vi "BioFeedback19(Adjustable_View).vi"() -> ()   [LabVIEW 2016]
doc: "Use this template to build a producer/consumer design pattern. Use this template when you need to execute a process, such as data analysis, when a data source, such as a triggered acquisition, produces data at an uneven rate and you need to execute the process when the data becomes available."
uses:
  customSubVIs/8ChanWfmArray.ctl
  <vilib>/Utility/file.llb/Write Delimited Spreadsheet (string).vi
  <vilib>/Waveform/WDTFileIO.llb/Export Waveforms To Spreadsheet File (1D).vi
panel:
  in  "log filepath":path
  out "TrialStartTime":timestamp
  in  "Trial Duration":dbl=3.0
  out "Trial Number":dbl
  in  "Session Name":string="Test"
  out "loopTime":dbl=30.0 caption="Upper Cut-Off"
  in  "trial display data":path
  out "Disp Data":cluster{"queue out":refnum<queue>, dbl, dbl}[](array[cluster])
  in  "Target Percentage":dbl=10.0
  out "DisplayActivation":dbl
  out "DisplayBarActivation":dbl(slide) caption="Percent Activation" max=1.0 scale=0.0..100.0
  in  "Display Channel":dbl=0.5
  out "MVC Data":cluster{"queue out":refnum<queue>, dbl, dbl}[](array[cluster])
  out "Trial Name":string="Test"
  in  "Data Directory":path=path "C:/Users/Tinggroup/Desktop/VRMuscleActivationVisualizer/LabviewFiles/Data"
  out "GetMaxStartTime":timestamp
  in  "MVC Number":dbl=1.0
  in  "SecondsToAcquireMax":dbl=3.0
  in  "Frames Per Second":dbl=30.0 caption="Upper Cut-Off"
  in  "EMG Input Device\nProduct Type":string="USB-6009"
  out "raw data":dynamicdata(graph)
  out "dispSize":dbl=20.0 caption="Lower Cut-Off"
  out "mvcSize":dbl=300.0 caption="Upper Cut-Off"
  in  "MVC Window Size (s)":dbl=0.5
  in  "Display Window Size (s)":dbl=0.5
  in  "MVC Raw Path":path
  in  "trial raw data":path
  in  "trial filtered data":path
  in  "MVC Filtered Path":path
  in  "Sample rate (Hz)":dbl=1000.0 caption="Upper Cut-Off"
  out "fps":dbl=20.0 caption="Lower Cut-Off"
  out "rate":dbl=300.0 caption="Upper Cut-Off"
  in  "Set Parameters":bool
  out "lower":dbl=20.0 caption="Lower Cut-Off"
  out "upper":dbl=300.0 caption="Upper Cut-Off"
  in  "Lower Cut-Off":dbl=20.0
  in  "Upper Cut-Off":dbl=500.0
  in  "Mark":bool
  in  "End Trial":bool
  in  "Reset MVC":bool
  in  "Get MVC":bool
  in  "StartTrial":bool
  out "State":T1(ring)
  out "FilteredAndRectified":waveform(dbl)[](graph) caption="Filtered and Rectified"
  in  "stop":bool
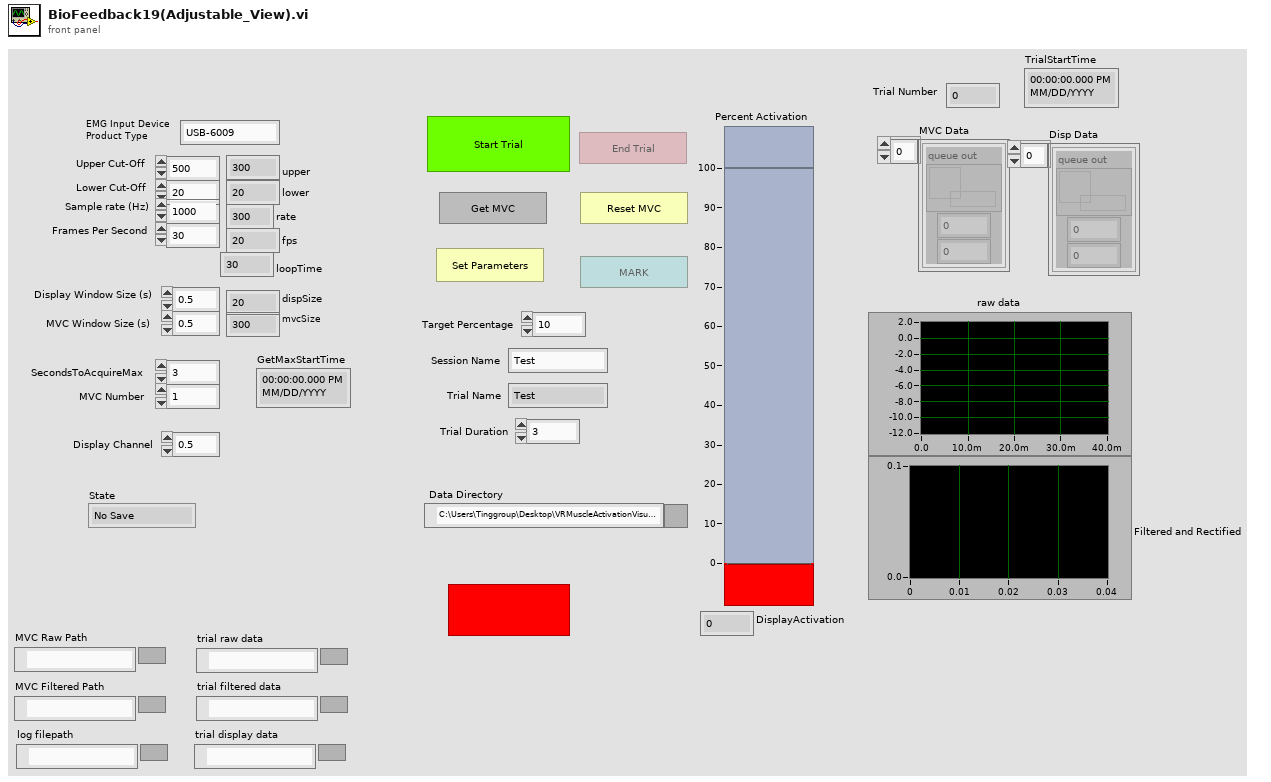
[diagram p1: front panel]
types:
  T1 = enum16{"No Save", "Acquiring Max", "Trial In Progress"}
  T2 = typedef "8ChanWfmArray.ctl" = waveform(dbl)[]
  T3 = enum8{"Enabled", "Disabled", "Disabled and Grayed Out"}
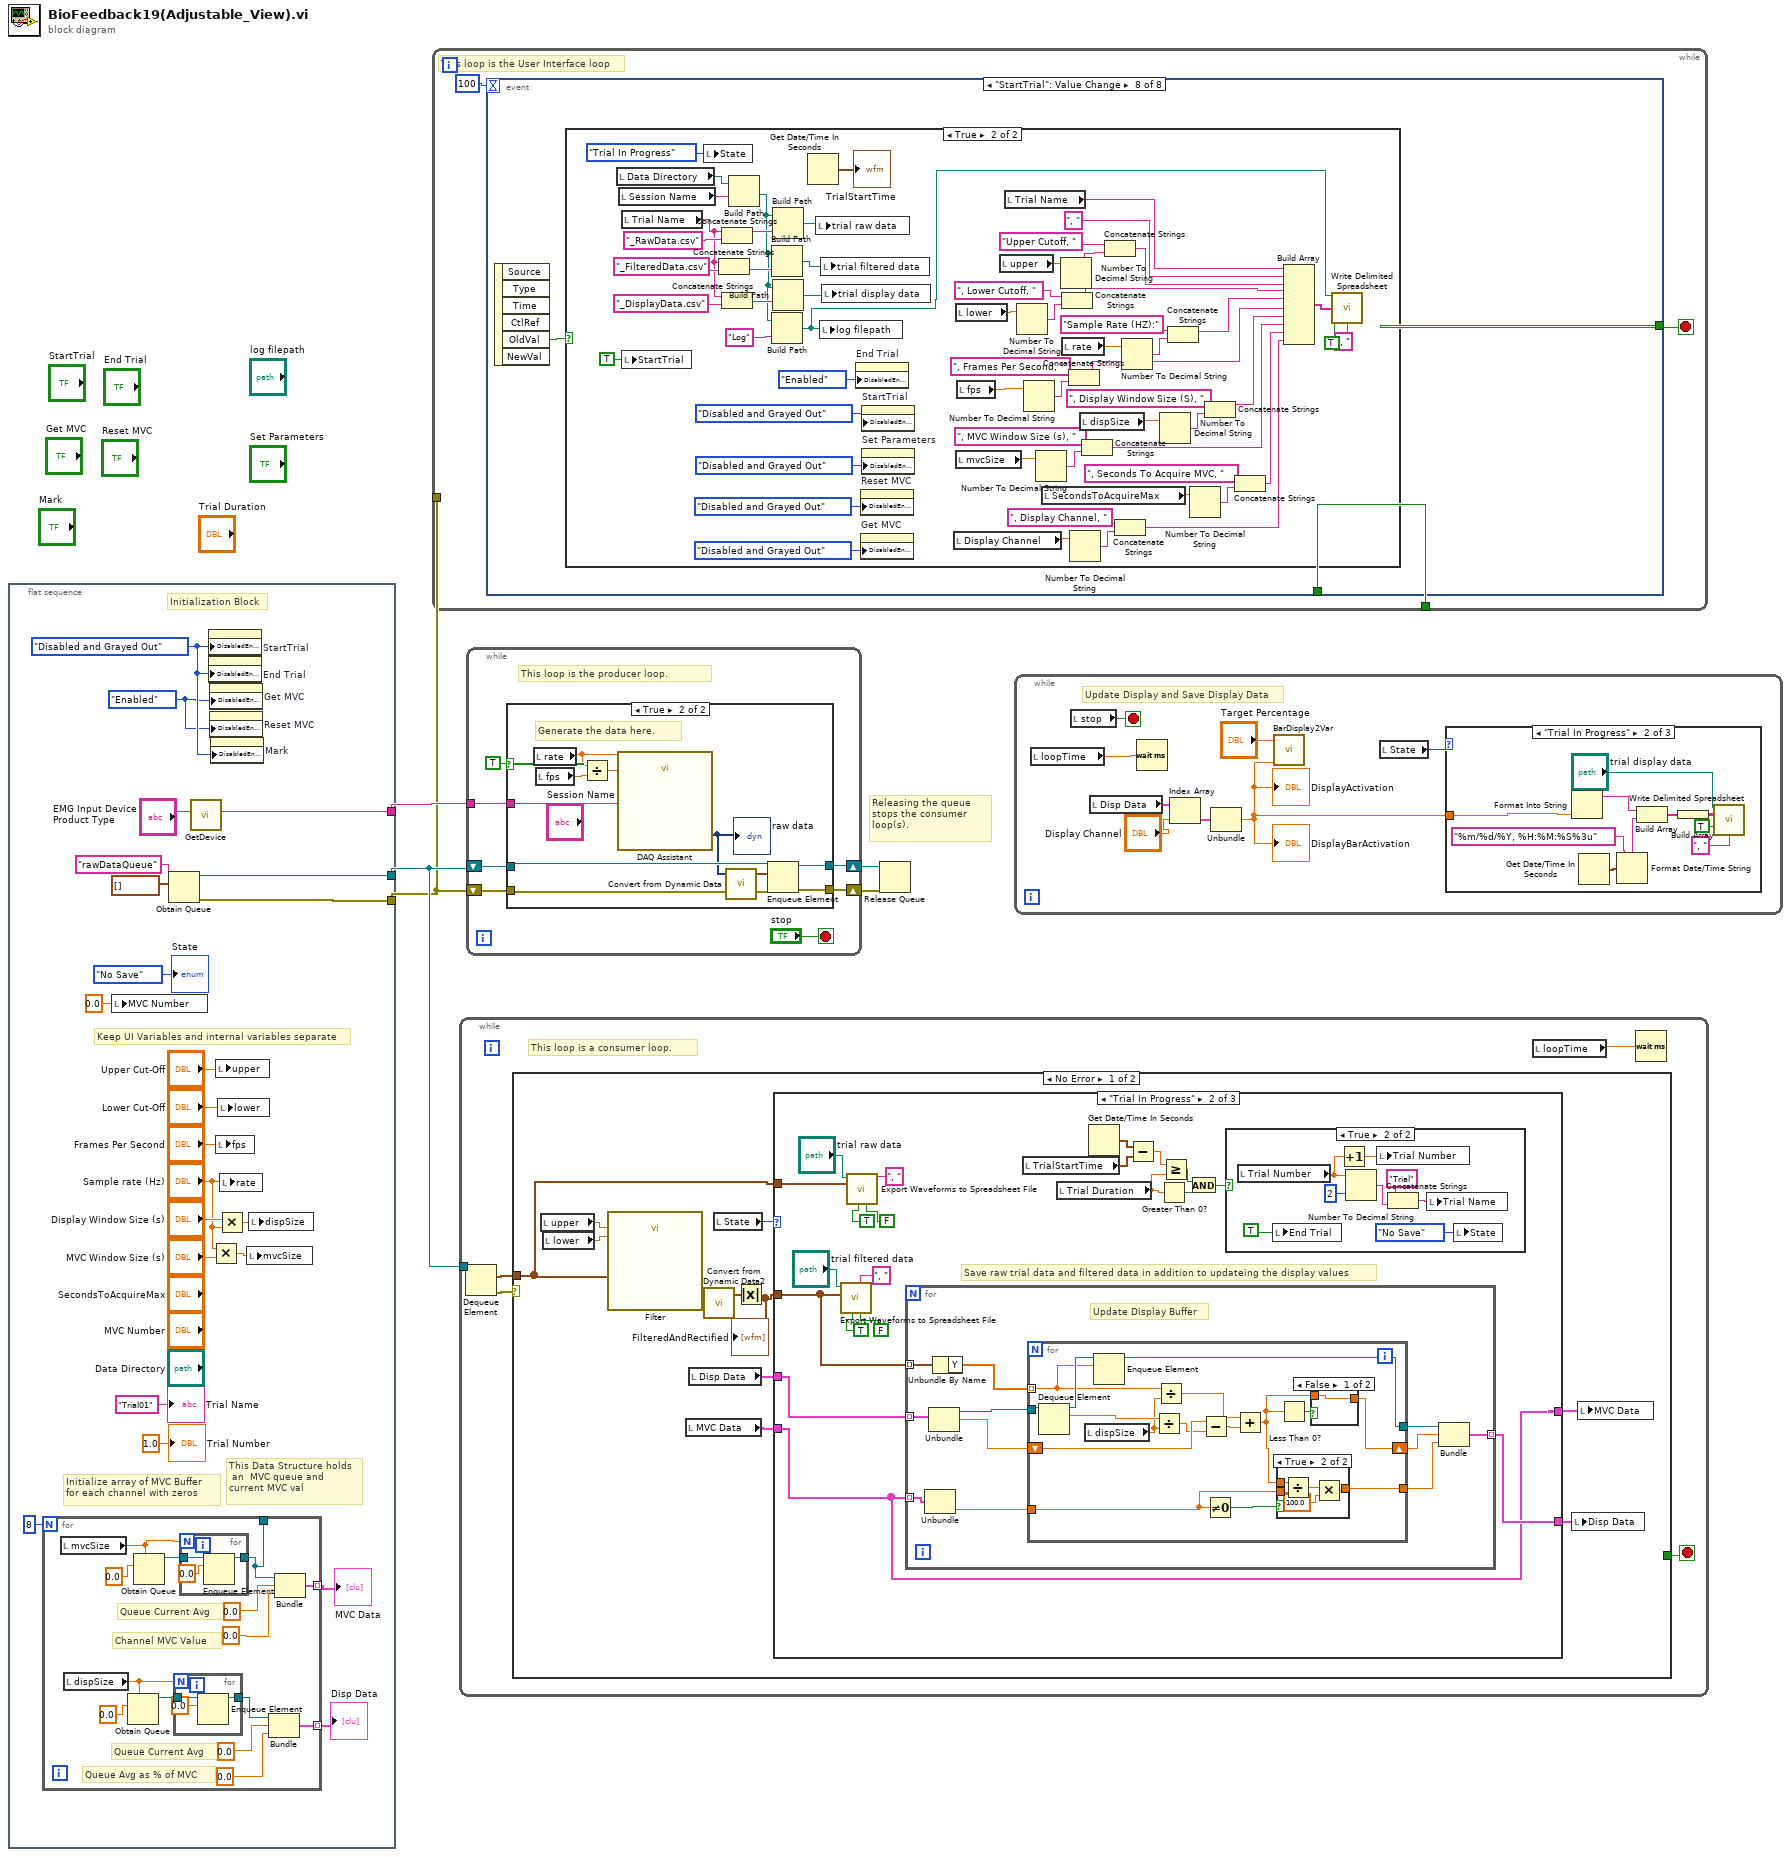
[diagram p0: block diagram]
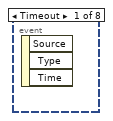
[diagram p4: hidden frame]
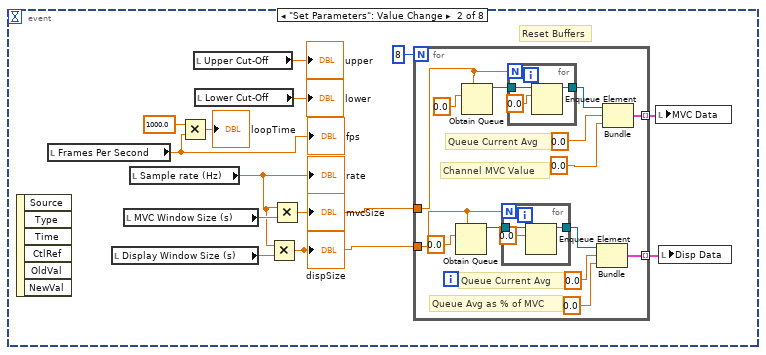
[diagram p5: hidden frame]
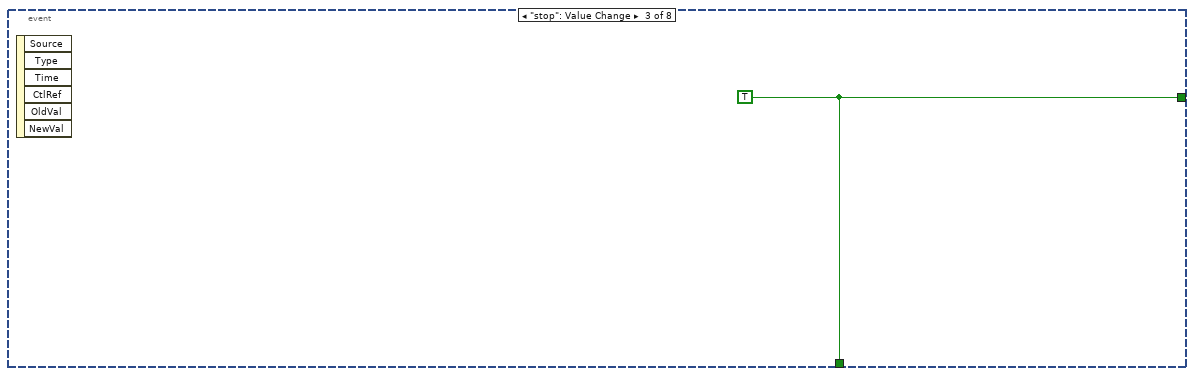
[diagram p6: hidden frame]
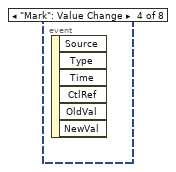
[diagram p7: hidden frame]
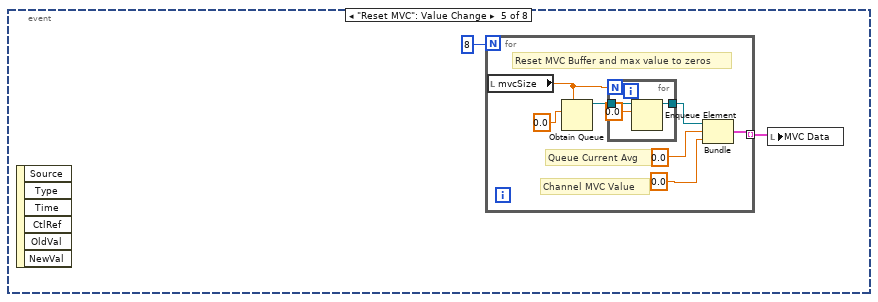
[diagram p8: hidden frame]
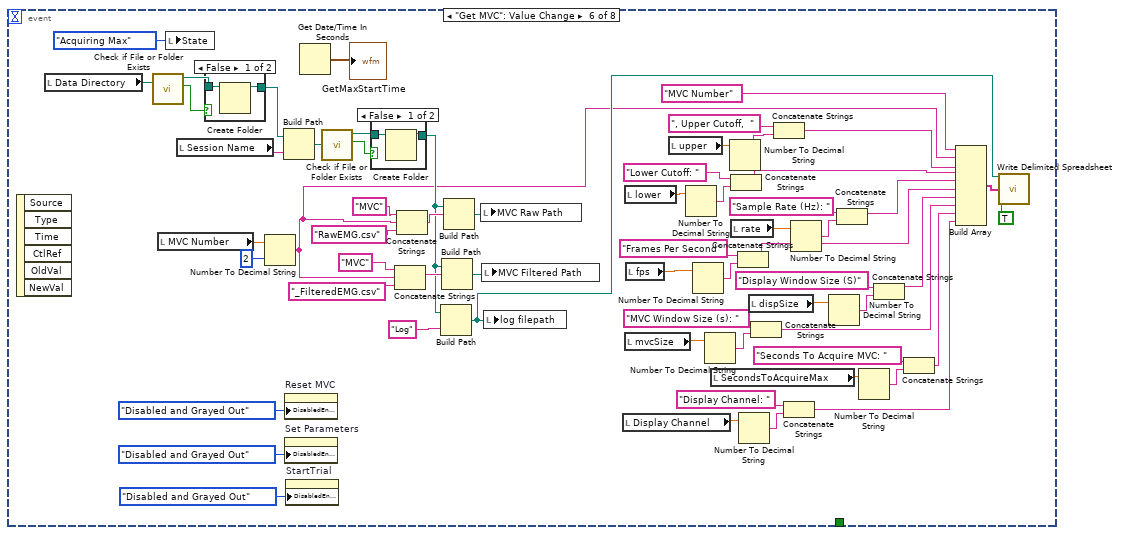
[diagram p9: hidden frame]
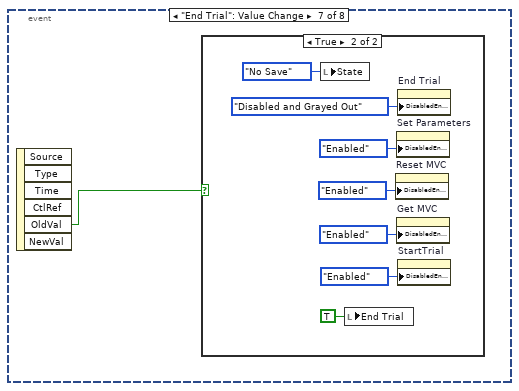
[diagram p12: hidden frame]
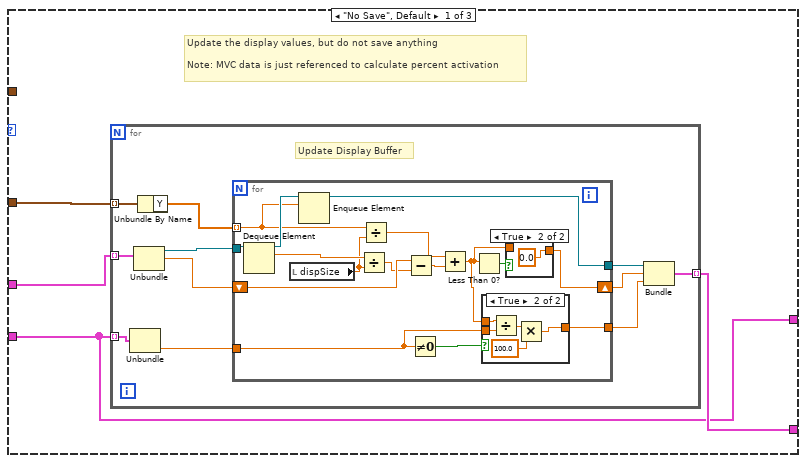
[diagram p15: hidden frame]
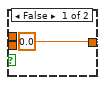
[diagram p17: hidden frame]
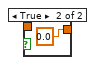
[diagram p19: hidden frame]
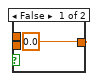
[diagram p20: hidden frame]
diagram:
  # "Releasing the queue stops the consumer loop(s)."
  n1 = flat-sequence {
    tunnel: [w19] -> w3
    tunnel: [w18] -> w2
    tunnel: [w21] -> w4
    frame #0 {
      w25 = T3."Enabled" ("Disabled")
      w26 = T3."Disabled and Grayed Out" ("Disabled")
      # "Keep UI Variables and internal variables separate"
      # "This Data Structure holds\n an  MVC queue and \ncurrent MVC val"
      # "Initialize array of MVC Buffer \nfor each channel with zeros"
      # "Initialization Block"
      n2 = for {
        N: 8 -> [_]
        tunnel: [w39] -> w11 mode=indexing
        tunnel: [w36] -> _
        tunnel: [w29] -> w10 mode=indexing
        # "Queue Avg as % of MVC"
        # "Queue Current Avg"
        # "Channel MVC Value"
        # "Queue Current Avg"
        n3 = local read "mvcSize"() -> (w40:dbl)
        n4 = local read "dispSize"() -> (w33:dbl)
        n5 = Obtain Queue(max queue size (-1, unlimited)=w33, element data type=0.0) -> (queue out=w30:refnum<queue>)  [unwired: 3 in, 2 out]
        n6 = Obtain Queue(max queue size (-1, unlimited)=w40, element data type=0.0) -> (queue out=w41:refnum<queue>)  [unwired: 3 in, 2 out]
        n7 = for {
          N: w33 -> [_]
          tunnel: w30 -> [w45]
          tunnel: [w43] -> w31
          n8 = Enqueue Element(queue=w45, element=0.0) -> (queue out=w43:refnum<queue>)  [unwired: 2 in, 2 out]
        }
        n9 = for {
          N: w40 -> [_]
          tunnel: w41 -> [w48]
          tunnel: [w46] -> w36
          n10 = Enqueue Element(queue=w48, element=0.0) -> (queue out=w46:refnum<queue>)  [unwired: 2 in, 2 out]
        }
        n11 = Bundle("queue out"=w31, 0.0, 0.0) -> (w29:cluster{"queue out":refnum<queue>, dbl, dbl})  [unwired: 1 in]
        n12 = Bundle("queue out"=w36, 0.0, 0.0) -> (w39:cluster{"queue out":refnum<queue>, dbl, dbl})  [unwired: 1 in]
      }
      "MVC Data" <- w11
      "Disp Data" <- w10
      n13 = local write "MVC Number"(0.0 ("MVC Number")) -> ()
      n14 = Obtain Queue(name (unnamed)="rawDataQueue", element data type=T2 [] ("initialized array")) -> (queue out=w19:refnum<queue>, error out=w18:errorcluster)  [unwired: 3 in, 1 out]
      n15 = call "GetDevice.vi"("EMG Input Device\nProduct Type"="EMG Input Device\nProduct Type") -> ("DAQmx Device Name"=w21:tag)  [unwired: 10 in]
      n16 = property on="StartTrial" class="Bool (strict)"("DisabledEnum"=w26) -> ()  [unwired: 2 in, 2 out]
      n17 = property on="End Trial" class="Bool (strict)"("DisabledEnum"=w26) -> ()  [unwired: 2 in, 2 out]
      n18 = property on="Get MVC" class="Bool"("DisabledEnum"=w25) -> ()  [unwired: 2 in, 2 out]
      n19 = property on="Reset MVC" class="Bool"("DisabledEnum"=w25) -> ()  [unwired: 2 in, 2 out]
      n20 = property on="Mark" class="Bool"("DisabledEnum"=w26) -> ()  [unwired: 2 in, 2 out]
      n21 = Multiply(x="Sample rate (Hz)", y="MVC Window Size (s)") -> (x*y=w13:dbl)
      n22 = local write "upper"("Upper Cut-Off") -> ()
      n23 = local write "fps"("Frames Per Second") -> ()
      n24 = Multiply(x="Display Window Size (s)", y="Sample rate (Hz)") -> (x*y=w16:dbl)
      n25 = local write "lower"("Lower Cut-Off") -> ()
      n26 = local write "rate"("Sample rate (Hz)") -> ()
      n27 = local write "mvcSize"(w13) -> ()
      n28 = local write "dispSize"(w16) -> ()
      "Trial Name" <- "Trial01" ("Trial Name")
      "State" <- T1."No Save" ("State")
      "Trial Number" <- 1.0 ("Trial Number")
    }
  }
  n29 = while {
    tunnel: [w51] -> _
    tunnel: w2 -> [_]
    stop <- w49 stop-if-true
    # "This loop is the User Interface loop"
    n30 = event shown="[7] \"StartTrial\": Value Change" {
      selector: _ -> [_ _ _ _ _ _ _ _]
      dyn-events: _ -> [_ _ _ _ _ _ _ _]
      timeout: u32 100 ("milliseconds to wait") -> [_ _ _ _ _ _ _ _]
      tunnel: [_ _ w85 _ _ _ _ _] -> w49
      tunnel: [_ _ w85 _ _ _ _ _] -> w51
      event Timeout {
        n31 = event-data() -> ()  [unwired: 1 in, 3 out]
      }
      event "Set Parameters": Value Change {
        # "Reset Buffers"
        n32 = event-data() -> ()  [unwired: 1 in, 6 out]
        n33 = local read "Frames Per Second"() -> (w52:dbl)
        "fps" <- w52
        n34 = local read "Display Window Size (s)"() -> (w62:dbl)
        n35 = local read "MVC Window Size (s)"() -> (w63:dbl)
        n36 = local read "Sample rate (Hz)"() -> (w60:dbl)
        "rate" <- w60
        n37 = Multiply(x=1000.0, y=w52) -> (x*y=→"loopTime":dbl)
        n38 = local read "Upper Cut-Off"() -> (→"upper":dbl)
        n39 = local read "Lower Cut-Off"() -> (→"lower":dbl)
        n40 = Multiply(x=w60, y=w62) -> (x*y=w58:dbl)
        "dispSize" <- w58
        n41 = Multiply(x=w60, y=w63) -> (x*y=w59:dbl)
        "mvcSize" <- w59
        n42 = for {
          N: 8 -> [_]
          tunnel: [w76] -> w56 mode=indexing
          tunnel: [w67] -> w57 mode=indexing
          tunnel: w59 -> [w66]
          tunnel: w58 -> [w65]
          # "Queue Avg as % of MVC"
          # "Queue Current Avg"
          # "Channel MVC Value"
          # "Queue Current Avg"
          n43 = Obtain Queue(max queue size (-1, unlimited)=w65, element data type=0.0) -> (queue out=w68:refnum<queue>)  [unwired: 3 in, 2 out]
          n44 = Obtain Queue(max queue size (-1, unlimited)=w66, element data type=0.0) -> (queue out=w77:refnum<queue>)  [unwired: 3 in, 2 out]
          n45 = for {
            N: w65 -> [_]
            tunnel: w68 -> [w81]
            tunnel: [w79] -> w69
            n46 = Enqueue Element(queue=w81, element=0.0) -> (queue out=w79:refnum<queue>)  [unwired: 2 in, 2 out]
          }
          n47 = for {
            N: w66 -> [_]
            tunnel: w77 -> [w84]
            tunnel: [w82] -> w73
            n48 = Enqueue Element(queue=w84, element=0.0) -> (queue out=w82:refnum<queue>)  [unwired: 2 in, 2 out]
          }
          n49 = Bundle("queue out"=w69, 0.0, 0.0) -> (w67:cluster{"queue out":refnum<queue>, dbl, dbl})  [unwired: 1 in]
          n50 = Bundle("queue out"=w73, 0.0, 0.0) -> (w76:cluster{"queue out":refnum<queue>, dbl, dbl})  [unwired: 1 in]
        }
        n51 = local write "MVC Data"(w56) -> ()
        n52 = local write "Disp Data"(w57) -> ()
      }
      event "stop": Value Change {
        w85 = TRUE
        n53 = event-data() -> ()  [unwired: 1 in, 6 out]
      }
      event "Mark": Value Change {
        n54 = event-data() -> ()  [unwired: 1 in, 6 out]
      }
      event "Reset MVC": Value Change {
        n55 = event-data() -> ()  [unwired: 1 in, 6 out]
        n56 = for {
          N: 8 -> [_]
          tunnel: [w88] -> w87 mode=indexing
          # "Channel MVC Value"
          # "Queue Current Avg"
          # "Reset MVC Buffer and max value to zeros"
          n57 = local read "mvcSize"() -> (w91:dbl)
          n58 = Obtain Queue(max queue size (-1, unlimited)=w91, element data type=0.0) -> (queue out=w90:refnum<queue>)  [unwired: 3 in, 2 out]
          n59 = for {
            N: w91 -> [_]
            tunnel: w90 -> [w97]
            tunnel: [w95] -> w92
            n60 = Enqueue Element(queue=w97, element=0.0) -> (queue out=w95:refnum<queue>)  [unwired: 2 in, 2 out]
          }
          n61 = Bundle("queue out"=w92, 0.0, 0.0) -> (w88:cluster{"queue out":refnum<queue>, dbl, dbl})  [unwired: 1 in]
        }
        n62 = local write "MVC Data"(w87) -> ()
      }
      event "Get MVC": Value Change {
        n63 = event-data() -> ()  [unwired: 1 in, 6 out]
        n64 = local read "Data Directory"() -> (w148:path)
        n65 = call <vilib>:"Check if File or Folder Exists.vi"("path"=w148) -> ("file or folder exists?"=w145:bool, "dup path"=w152:path)  [unwired: 8 in, 1 out]
        n66 = local read "MVC Number"() -> (w151:dbl)
        n67 = local write "State"(T1."Acquiring Max" ("State")) -> ()
        n68 = local read "Session Name"() -> (w150:string)
        n69 = case shown="False" w145 {
          tunnel: w152 -> [w164 w165]
          tunnel: [w163 w165] -> w144
          frame False {
            n70 = Create Folder(path (use dialog)=w164) -> (created path=w163:path)  [unwired: 2 in, 2 out]
          }
          frame True {
          }
        }
        n71 = Number To Decimal String(number=w151, width (-)=i16 2) -> (decimal integer string=w99:string)
        n72 = Build Path(base path=w144, name or relative path=w150) -> (appended path=w149:path)
        n73 = property on="Reset MVC" class="Bool"("DisabledEnum"=T3."Disabled and Grayed Out" ("Disabled")) -> ()  [unwired: 2 in, 2 out]
        n74 = property on="Set Parameters" class="Bool"("DisabledEnum"=T3."Disabled and Grayed Out" ("Disabled")) -> ()  [unwired: 2 in, 2 out]
        n75 = property on="StartTrial" class="Bool (strict)"("DisabledEnum"=T3."Disabled and Grayed Out" ("Disabled")) -> ()  [unwired: 2 in, 2 out]
        n76 = Get Date/Time In Seconds() -> (seconds since 1Jan1904=→"GetMaxStartTime":timestamp)
        n77 = call <vilib>:"Check if File or Folder Exists.vi"("path"=w149) -> ("file or folder exists?"=w147:bool, "dup path"=w146:path)  [unwired: 8 in, 1 out]
        n78 = case shown="False" w147 {
          tunnel: w146 -> [w161 w162]
          tunnel: [w160 w162] -> w135
          frame False {
            n79 = Create Folder(path (use dialog)=w161) -> (created path=w160:path)  [unwired: 2 in, 2 out]
          }
          frame True {
          }
        }
        n80 = Concatenate Strings("MVC" ("string"), w99, "_FilteredEMG.csv" ("string")) -> (w157:string)
        n81 = Concatenate Strings("MVC" ("string"), w99, "RawEMG.csv" ("string")) -> (w156:string)
        n82 = Build Path(base path=w135, name or relative path="Log" ("string")) -> (appended path=w101:path)
        n83 = Build Path(base path=w135, name or relative path=w157) -> (appended path=w142:path)
        n84 = Build Path(base path=w135, name or relative path=w156) -> (appended path=w141:path)
        n85 = local write "MVC Raw Path"(w141) -> ()
        n86 = local write "MVC Filtered Path"(w142) -> ()
        n87 = local write "log filepath"(w101) -> ()
        n88 = local read "Display Channel"() -> (w104:dbl)
        n89 = local read "lower"() -> (w129:dbl)
        n90 = local read "mvcSize"() -> (w112:dbl)
        n91 = local read "fps"() -> (w122:dbl)
        n92 = local read "upper"() -> (w134:dbl)
        n93 = Number To Decimal String(number=w129) -> (decimal integer string=w130:string)  [unwired: 1 in]
        n94 = Number To Decimal String(number=w122) -> (decimal integer string=w123:string)  [unwired: 1 in]
        n95 = Number To Decimal String(number=w112) -> (decimal integer string=w113:string)  [unwired: 1 in]
        n96 = local read "SecondsToAcquireMax"() -> (w108:dbl)
        n97 = Number To Decimal String(number=w134) -> (decimal integer string=w132:string)  [unwired: 1 in]
        n98 = Concatenate Strings("Lower Cutoff: ", w130) -> (w121:string)
        n99 = local read "rate"() -> (w126:dbl)
        n100 = Concatenate Strings("Frames Per Second", w123) -> (w119:string)
        n101 = Number To Decimal String(number=w104) -> (decimal integer string=w105:string)  [unwired: 1 in]
        n102 = local read "dispSize"() -> (w116:dbl)
        n103 = Concatenate Strings("MVC Window Size (s): ", w113) -> (w111:string)
        n104 = Concatenate Strings(", Upper Cutoff,  ", w132) -> (w125:string)
        n105 = Concatenate Strings("Display Channel: ", w105) -> (w103:string)
        n106 = Number To Decimal String(number=w126) -> (decimal integer string=w127:string)  [unwired: 1 in]
        n107 = Number To Decimal String(number=w116) -> (decimal integer string=w117:string)  [unwired: 1 in]
        n108 = Concatenate Strings("Sample Rate (Hz): ", w127) -> (w120:string)
        n109 = Number To Decimal String(number=w108) -> (decimal integer string=w109:string)  [unwired: 1 in]
        n110 = Concatenate Strings("Display Window Size (S)", w117) -> (w115:string)
        n111 = Concatenate Strings("Seconds To Acquire MVC: ", w109) -> (w107:string)
        n112 = Build Array("MVC Number" ("element"), w99, w125, w121, w120, w119, w115, w111, w107, w103) -> (w102:string[])
        n113 = call-poly <vilib>:"Write Delimited Spreadsheet.vi"("file path (dialog if empty)"=w101, "1D data"=w102, "append to file? (new file:F)"=TRUE) -> ()  [unwired: 11 in, 2 out]
      }
      event "End Trial": Value Change {
        n114 = event-data() -> ("OldVal"=w166:bool)  [unwired: 1 in, 5 out]
        n115 = case shown="True" w166 {
          frame False {
          }
          frame True {
            n116 = local write "State"(T1."No Save" ("State")) -> ()
            n117 = local write "End Trial"(TRUE ("End Trial")) -> ()
            n118 = property on="Reset MVC" class="Bool"("DisabledEnum"=T3."Enabled" ("Disabled")) -> ()  [unwired: 2 in, 2 out]
            n119 = property on="Set Parameters" class="Bool"("DisabledEnum"=T3."Enabled" ("Disabled")) -> ()  [unwired: 2 in, 2 out]
            n120 = property on="Get MVC" class="Bool"("DisabledEnum"=T3."Enabled" ("Disabled")) -> ()  [unwired: 2 in, 2 out]
            n121 = property on="End Trial" class="Bool (strict)"("DisabledEnum"=T3."Disabled and Grayed Out" ("Disabled")) -> ()  [unwired: 2 in, 2 out]
            n122 = property on="StartTrial" class="Bool (strict)"("DisabledEnum"=T3."Enabled" ("Disabled")) -> ()  [unwired: 2 in, 2 out]
          }
        }
      }
      event "StartTrial": Value Change {
        n123 = event-data() -> ("OldVal"=w174:bool)  [unwired: 1 in, 5 out]
        n124 = case shown="True" w174 {
          frame False {
          }
          frame True {
            n125 = local read "Data Directory"() -> (w226:path)
            n126 = local read "Session Name"() -> (w225:string)
            n127 = local read "Trial Name"() -> (w183:string)
            n128 = local write "StartTrial"(TRUE ("StartTrial")) -> ()
            n129 = local write "State"(T1."Trial In Progress" ("State")) -> ()
            n130 = Concatenate Strings(w183, "_FilteredData.csv" ("string")) -> (w230:string)
            n131 = Concatenate Strings(w183, "_RawData.csv" ("string")) -> (w228:string)
            n132 = Concatenate Strings(w183, "_DisplayData.csv" ("string")) -> (w232:string)
            n133 = Build Path(base path=w226, name or relative path=w225) -> (appended path=w182:path)
            n134 = Build Path(base path=w182, name or relative path=w230) -> (appended path=w224:path)
            n135 = Build Path(base path=w182, name or relative path="Log" ("string")) -> (appended path=w180:path)
            n136 = Build Path(base path=w182, name or relative path=w228) -> (appended path=w223:path)
            n137 = Build Path(base path=w182, name or relative path=w232) -> (appended path=w233:path)
            n138 = Get Date/Time In Seconds() -> (seconds since 1Jan1904=→"TrialStartTime":timestamp)
            n139 = local write "trial raw data"(w223) -> ()
            n140 = local write "log filepath"(w180) -> ()
            n141 = local write "trial filtered data"(w224) -> ()
            n142 = local write "trial display data"(w233) -> ()
            n143 = property on="End Trial" class="Bool (strict)"("DisabledEnum"=T3."Enabled" ("Disabled")) -> ()  [unwired: 2 in, 2 out]
            n144 = property on="Reset MVC" class="Bool"("DisabledEnum"=T3."Disabled and Grayed Out" ("Disabled")) -> ()  [unwired: 2 in, 2 out]
            n145 = property on="Get MVC" class="Bool"("DisabledEnum"=T3."Disabled and Grayed Out" ("Disabled")) -> ()  [unwired: 2 in, 2 out]
            n146 = property on="StartTrial" class="Bool (strict)"("DisabledEnum"=T3."Disabled and Grayed Out" ("Disabled")) -> ()  [unwired: 2 in, 2 out]
            n147 = property on="Set Parameters" class="Bool"("DisabledEnum"=T3."Disabled and Grayed Out" ("Disabled")) -> ()  [unwired: 2 in, 2 out]
            n148 = local read "Display Channel"() -> (w215:dbl)
            n149 = local read "lower"() -> (w190:dbl)
            n150 = local read "mvcSize"() -> (w207:dbl)
            n151 = local read "fps"() -> (w197:dbl)
            n152 = local read "upper"() -> (w185:dbl)
            n153 = local read "Trial Name"() -> (w177:string)
            n154 = Number To Decimal String(number=w190) -> (decimal integer string=w189:string)  [unwired: 1 in]
            n155 = Number To Decimal String(number=w197) -> (decimal integer string=w196:string)  [unwired: 1 in]
            n156 = Number To Decimal String(number=w207) -> (decimal integer string=w206:string)  [unwired: 1 in]
            n157 = local read "SecondsToAcquireMax"() -> (w211:dbl)
            n158 = Number To Decimal String(number=w185) -> (decimal integer string=w187:string)  [unwired: 1 in]
            n159 = Concatenate Strings(", Lower Cutoff, ", w189) -> (w198:string)
            n160 = local read "rate"() -> (w193:dbl)
            n161 = Concatenate Strings(", Frames Per Second, ", w196) -> (w200:string)
            n162 = Number To Decimal String(number=w215) -> (decimal integer string=w214:string)  [unwired: 1 in]
            n163 = local read "dispSize"() -> (w203:dbl)
            n164 = Concatenate Strings(", MVC Window Size (s), ", w206) -> (w208:string)
            n165 = Concatenate Strings("Upper Cutoff, ", w187) -> (w194:string)
            n166 = Concatenate Strings(", Display Channel, ", w214) -> (w216:string)
            n167 = Number To Decimal String(number=w193) -> (decimal integer string=w192:string)  [unwired: 1 in]
            n168 = Number To Decimal String(number=w203) -> (decimal integer string=w202:string)  [unwired: 1 in]
            n169 = Concatenate Strings("Sample Rate (HZ):", w192) -> (w199:string)
            n170 = Number To Decimal String(number=w211) -> (decimal integer string=w210:string)  [unwired: 1 in]
            n171 = Concatenate Strings(", Display Window Size (S), ", w202) -> (w204:string)
            n172 = Concatenate Strings(", Seconds To Acquire MVC, ", w210) -> (w212:string)
            n173 = Build Array(w177, ", " ("element"), w194, w198, w199, w200, w204, w208, w212, w216) -> (w217:string[])
            n174 = call-poly <vilib>:"Write Delimited Spreadsheet.vi"("file path (dialog if empty)"=w180, "1D data"=w217, "append to file? (new file:F)"=TRUE, "delimiter (\\t)"=", " ("delimiter (\\t)")) -> ()  [unwired: 10 in, 2 out]
          }
        }
      }
    }
  }
  n175 = while {
    tunnel: w3 -> [w236]
    stop <- w237 stop-if-true
    # "This loop is a consumer loop."
    n176 = Dequeue Element(queue=w236) -> (element=w238:T2, error out=w239:errorcluster)  [unwired: 2 in, 2 out]
    n177 = case shown="No Error" w239 {
      tunnel: w238 -> [w245 _]
      tunnel: [_ TRUE] -> w237
      frame No Error {
        n178 = local read "upper"() -> (w248:dbl)
        n179 = local read "lower"() -> (w247:dbl)
        n180 = call "Filter"("Lower Cut-Off"=w247, "Upper Cut-Off"=w248, "Signal"=w245) -> ("Filtered Signal"=w249:dynamicdata)  [unwired: 7 in, 1 out]
        n181 = local read "MVC Data"() -> (w243:cluster{"queue out":refnum<queue>, dbl, dbl}[])
        n182 = local read "Disp Data"() -> (w242:cluster{"queue out":refnum<queue>, dbl, dbl}[])
        n183 = call "Convert from Dynamic Data2"("Dynamic Data Type"=w249) -> ("Array of Waveform"=w250:waveform(dbl)[])  [unwired: 3 in]
        n184 = local read "State"() -> (w246:T1)
        n185 = Absolute Value(x=w250) -> (abs(x)=w244:waveform(dbl)[])
        "FilteredAndRectified" <- w244
        n186 = case shown="\"Trial In Progress\"" w246 {
          tunnel: w244 -> [w254 w301 w365]
          tunnel: w245 -> [_ w304 w366]
          tunnel: w243 -> [w251 w299 w356]
          tunnel: w242 -> [w253 w302 w355]
          tunnel: [w252 w300 w357] -> w240
          tunnel: [w251 w299 w358] -> w241
          frame "No Save", Default {
            # "Update the display values, but do not save anything\n\nNote: MVC data is just referenced to calculate percent activation"
            n187 = for {
              tunnel: w253 -> [w259] mode=indexing
              tunnel: w254 -> [w264] mode=indexing
              tunnel: [w260] -> w252 mode=indexing
              tunnel: w251 -> [w257] mode=indexing
              # "Update Display Buffer"
              n188 = Unbundle(w257) -> (w256:dbl)  [unwired: 2 out]
              n189 = Unbundle(w259) -> ("queue out"=w265:refnum<queue>, w258:dbl)  [unwired: 1 out]
              n190 = Unbundle By Name(w264) -> ("Y"=w263:dbl[])
              n191 = for {
                tunnel: w265 -> [w275]
                tunnel: w263 -> [w271] mode=indexing
                shift-right: [w268] -> w262
                shift-left: w258 -> [w280]
                tunnel: [w270] -> w261
                tunnel: w256 -> [w273]
                tunnel: [w269] -> w255
                n192 = Dequeue Element(queue=w275) -> (queue out=w272:refnum<queue>, element=w281:dbl)  [unwired: 2 in, 2 out]
                n193 = local read "dispSize"() -> (w278:dbl)
                n194 = Enqueue Element(queue=w272, element=w271) -> (queue out=w270:refnum<queue>)  [unwired: 2 in, 2 out]
                n195 = Divide(x=w281, y=w278) -> (x/y=w279:dbl)
                n196 = Divide(x=w271, y=w278) -> (x/y=w276:dbl)
                n197 = Subtract(x=w280, y=w279) -> (x-y=w277:dbl)
                n198 = Not Equal To 0?(x=w273) -> (x != 0?=w274:bool)
                n199 = Add(x=w276, y=w277) -> (x+y=w266:dbl)
                n200 = Less Than 0?(x=w266) -> (x < 0?=w267:bool)
                n201 = case shown="True" w274 {
                  tunnel: w273 -> [_ w289]
                  tunnel: [0.0 w285] -> w269
                  tunnel: w266 -> [_ w288]
                  frame False {
                  }
                  frame True {
                    n202 = Divide(x=w288, y=w289) -> (x/y=w286:dbl)
                    n203 = Multiply(x=w286, y=100.0) -> (x*y=w285:dbl)
                  }
                }
                n204 = case shown="True" w267 {
                  tunnel: [w282 0.0] -> w268
                  tunnel: w266 -> [w282 _]
                  frame False {
                  }
                  frame True {
                  }
                }
              }
              n205 = Bundle("queue out"=w261, w262, w255) -> (w260:cluster{"queue out":refnum<queue>, dbl, dbl})  [unwired: 1 in]
            }
          }
          frame "Trial In Progress" {
            # "Save raw trial data and filtered data in addition to updateing the display values"
            n206 = call-poly <vilib>:"Export Waveforms to Spreadsheet File.vi"("header? (write header:T)"=FALSE, "delimiter (Tab)"=", ", "append to file? (new file:F)"=TRUE, "waveforms"=w301, "file path (dialog if empty)"="trial filtered data") -> ()  [unwired: 5 in, 2 out]
            n207 = call-poly <vilib>:"Export Waveforms to Spreadsheet File.vi"("header? (write header:T)"=FALSE, "delimiter (Tab)"=", ", "append to file? (new file:F)"=TRUE, "waveforms"=w304, "file path (dialog if empty)"="trial raw data") -> ()  [unwired: 5 in, 2 out]
            n208 = for {
              tunnel: w302 -> [w322] mode=indexing
              tunnel: w301 -> [w327] mode=indexing
              tunnel: [w323] -> w300 mode=indexing
              tunnel: w299 -> [w320] mode=indexing
              # "Update Display Buffer"
              n209 = Unbundle(w320) -> (w319:dbl)  [unwired: 2 out]
              n210 = Unbundle(w322) -> ("queue out"=w328:refnum<queue>, w321:dbl)  [unwired: 1 out]
              n211 = Unbundle By Name(w327) -> ("Y"=w326:dbl[])
              n212 = for {
                tunnel: w328 -> [w338]
                tunnel: w326 -> [w334] mode=indexing
                shift-right: [w329] -> w325
                shift-left: w321 -> [w343]
                tunnel: [w333] -> w324
                tunnel: w319 -> [w336]
                tunnel: [w332] -> w318
                n213 = Dequeue Element(queue=w338) -> (queue out=w335:refnum<queue>, element=w344:dbl)  [unwired: 2 in, 2 out]
                n214 = local read "dispSize"() -> (w341:dbl)
                n215 = Enqueue Element(queue=w335, element=w334) -> (queue out=w333:refnum<queue>)  [unwired: 2 in, 2 out]
                n216 = Divide(x=w344, y=w341) -> (x/y=w342:dbl)
                n217 = Divide(x=w334, y=w341) -> (x/y=w339:dbl)
                n218 = Subtract(x=w343, y=w342) -> (x-y=w340:dbl)
                n219 = Not Equal To 0?(x=w336) -> (x != 0?=w337:bool)
                n220 = Add(x=w339, y=w340) -> (x+y=w330:dbl)
                n221 = case shown="True" w337 {
                  tunnel: w336 -> [_ w352]
                  tunnel: [0.0 w350] -> w332
                  tunnel: w330 -> [_ w351]
                  frame False {
                  }
                  frame True {
                    n222 = Divide(x=w351, y=w352) -> (x/y=w349:dbl)
                    n223 = Multiply(x=w349, y=100.0) -> (x*y=w350:dbl)
                  }
                }
                n224 = Less Than 0?(x=w330) -> (x < 0?=w331:bool)
                n225 = case shown="False" w331 {
                  tunnel: [w345 0.0] -> w329
                  tunnel: w330 -> [w345 _]
                  frame False {
                  }
                  frame True {
                  }
                }
              }
              n226 = Bundle("queue out"=w324, w325, w318) -> (w323:cluster{"queue out":refnum<queue>, dbl, dbl})  [unwired: 1 in]
            }
            n227 = local read "TrialStartTime"() -> (w295:timestamp)
            n228 = local read "Trial Duration"() -> (w291:dbl)
            n229 = Get Date/Time In Seconds() -> (seconds since 1Jan1904=w294:timestamp)
            n230 = Subtract(x=w294, y=w295) -> (x-y=w296:dbl)
            n231 = Greater Than 0?(x=w291) -> (x > 0?=w292:bool)
            n232 = Greater Or Equal?(x=w296, y=w291) -> (x >= y?=w290:bool)
            n233 = And(x=w290, y=w292) -> (x .and. y?=w293:bool)
            n234 = case shown="True" w293 {
              frame False {
              }
              frame True {
                n235 = local read "Trial Number"() -> (w314:dbl)
                n236 = local write "End Trial"(TRUE ("End Trial")) -> ()
                n237 = Increment(x=w314) -> (x+1=w317:dbl)
                n238 = Number To Decimal String(number=w314, width (-)=i16 2) -> (decimal integer string=w310:string)
                n239 = local write "Trial Number"(w317) -> ()
                n240 = Concatenate Strings("Trial" ("string"), w310) -> (w313:string)
                n241 = local write "Trial Name"(w313) -> ()
                n242 = local write "State"(T1."No Save" ("State")) -> ()
              }
            }
          }
          frame "Acquiring Max" {
            # "Automatically Stop Listening for Max after Acquire Max Time is elapsed"
            n243 = call-poly <vilib>:"Export Waveforms to Spreadsheet File.vi"("header? (write header:T)"=FALSE, "delimiter (Tab)"=", ", "append to file? (new file:F)"=TRUE, "waveforms"=w365, "file path (dialog if empty)"="MVC Filtered Path") -> ()  [unwired: 5 in, 2 out]
            n244 = call-poly <vilib>:"Export Waveforms to Spreadsheet File.vi"("header? (write header:T)"=FALSE, "delimiter (Tab)"=", ", "append to file? (new file:F)"=TRUE, "waveforms"=w366, "file path (dialog if empty)"="MVC Raw Path") -> ()  [unwired: 5 in, 2 out]
            n245 = for {
              tunnel: w365 -> [w392] mode=indexing
              tunnel: w356 -> [w390] mode=indexing
              tunnel: [w384] -> w358 mode=indexing
              tunnel: w355 -> [w382] mode=indexing
              tunnel: [w376] -> w357 mode=indexing
              # "For each channel, update Moving Average for each channel"
              n246 = Unbundle(w390) -> ("queue out"=w383:refnum<queue>, w389:dbl, w388:dbl)
              n247 = Unbundle By Name(w392) -> ("Y"=w391:dbl[])
              n248 = Unbundle(w382) -> ("queue out"=w378:refnum<queue>, w381:dbl)  [unwired: 1 out]
              n249 = for {
                tunnel: w391 -> [w401] mode=indexing
                shift-right: [w406] -> w386
                shift-left: w389 -> [w418]
                shift-right: [w410] -> w387
                shift-left: w383 -> [w409]
                shift-right: [w412] -> w385
                shift-left: w388 -> [w411]
                tunnel: w381 -> [w399]
                shift-right: [w394] -> w379
                shift-left: _ -> [_]
                shift-right: [w403] -> w380
                shift-left: w378 -> [w396]
                # "Update Max if necessary"
                # "Update MVC queue current avg and \nmax value for each data point"
                n250 = Dequeue Element(queue=w396) -> (queue out=w405:refnum<queue>, element=w404:dbl)  [unwired: 2 in, 2 out]
                n251 = local read "dispSize"() -> (w402:dbl)
                n252 = Dequeue Element(queue=w409) -> (queue out=w408:refnum<queue>, element=w407:dbl)  [unwired: 2 in, 2 out]
                n253 = Enqueue Element(queue=w405, element=w401) -> (queue out=w403:refnum<queue>)  [unwired: 2 in, 2 out]
                n254 = local read "mvcSize"() -> (w416:dbl)
                n255 = Divide(x=w404, y=w402) -> (x/y=w400:dbl)
                n256 = Enqueue Element(queue=w408, element=w401) -> (queue out=w410:refnum<queue>)  [unwired: 2 in, 2 out]
                n257 = Divide(x=w401, y=w402) -> (x/y=w398:dbl)
                n258 = Subtract(x=w399, y=w400) -> (x-y=w397:dbl)
                n259 = Divide(x=w407, y=w416) -> (x/y=w417:dbl)
                n260 = Divide(x=w401, y=w416) -> (x/y=w414:dbl)
                n261 = Add(x=w398, y=w397) -> (x+y=w393:dbl)
                n262 = Subtract(x=w418, y=w417) -> (x-y=w415:dbl)
                n263 = Add(x=w414, y=w415) -> (x+y=w406:dbl)
                n264 = Less Than 0?(x=w393) -> (x < 0?=w395:bool)
                n265 = Greater?(x=w406, y=w411) -> (0:w413:bool)
                n266 = case shown="True" w395 {
                  tunnel: [w419 0.0] -> w394
                  tunnel: w393 -> [w419 _]
                  frame False {
                  }
                  frame True {
                  }
                }
                n267 = case shown="False" w413 {
                  tunnel: w406 -> [_ w422]
                  tunnel: [w421 w422] -> w412
                  tunnel: w411 -> [w421 _]
                  frame False {
                  }
                  frame True {
                  }
                }
              }
              n268 = Bundle("queue out"=w380, w379, 0.0) -> (w376:cluster{"queue out":refnum<queue>, dbl, dbl})  [unwired: 1 in]
              n269 = Bundle("queue out"=w387, w386, w385) -> (w384:cluster{"queue out":refnum<queue>, dbl, dbl})  [unwired: 1 in]
            }
            n270 = local read "GetMaxStartTime"() -> (w362:timestamp)
            n271 = local read "SecondsToAcquireMax"() -> (w360:dbl)
            n272 = Get Date/Time In Seconds() -> (seconds since 1Jan1904=w363:timestamp)
            n273 = Subtract(x=w363, y=w362) -> (x-y=w361:dbl)
            n274 = Greater Or Equal?(x=w361, y=w360) -> (x >= y?=w359:bool)
            n275 = case shown="True" w359 {
              frame False {
              }
              frame True {
                w372 = T3."Enabled" ("Disabled")
                n276 = local read "MVC Number"() -> (w375:dbl)
                n277 = property on="StartTrial" class="Bool (strict)"("DisabledEnum"=w372) -> ()  [unwired: 2 in, 2 out]
                n278 = property on="Reset MVC" class="Bool"("DisabledEnum"=w372) -> ()  [unwired: 2 in, 2 out]
                n279 = property on="Set Parameters" class="Bool"("DisabledEnum"=w372) -> ()  [unwired: 2 in, 2 out]
                n280 = Increment(x=w375) -> (x+1=w374:dbl)
                n281 = local write "MVC Number"(w374) -> ()
                n282 = local write "State"(T1."No Save" ("State")) -> ()
              }
            }
          }
        }
        n283 = local write "Disp Data"(w240) -> ()
        n284 = local write "MVC Data"(w241) -> ()
      }
      frame Error {
        # "Return true for any case which should stop the loop."
      }
    }
    n285 = local read "loopTime"() -> (w235:dbl)
    n286 = Wait (ms)(milliseconds to wait=w235) -> ()  [unwired: 1 out]
  }
  n287 = while {
    shift-right: [w426] -> w1
    shift-left: w2 -> [w427]
    shift-right: [w428] -> w5
    shift-left: w3 -> [w429]
    tunnel: w4 -> [w424]
    stop <- "stop" stop-if-true
    # "This loop is the producer loop."
    n288 = case shown="True" TRUE ("Case Constant\n(See Context Help)") {
      tunnel: w429 -> [w432 w442]
      tunnel: [w432 w441] -> w428
      tunnel: w427 -> [w431 w440]
      tunnel: [w431 w439] -> w426
      tunnel: w424 -> [_ w433]
      frame False {
      }
      frame True {
        # "Generate the data here."
        n289 = local read "rate"() -> (w436:dbl)
        n290 = local read "fps"() -> (w437:dbl)
        n291 = Divide(x=w436, y=w437) -> (x/y=w435:dbl)
        n292 = call "DAQ Assistant"("rate"=w436, "number of samples"=w435, "device name"=w433) -> ("data"=w434:dynamicdata)  [unwired: 13 in, 3 out]
        "raw data" <- w434
        n293 = call "Convert from Dynamic Data"("Dynamic Data Type"=w434) -> ("Array of Waveform"=w438:waveform(dbl)[])  [unwired: 3 in]
        n294 = Enqueue Element(queue=w442, element=w438, error in (no error)=w440) -> (queue out=w441:refnum<queue>, error out=w439:errorcluster)  [unwired: 1 in, 1 out]
      }
    }
  }
  n295 = Release Queue(queue=w5, error in (no error)=w1) -> ()  [unwired: 1 in, 3 out]
  n296 = while {
    stop <- w446 stop-if-true
    # "Update Display and Save Display Data"
    n297 = local read "loopTime"() -> (w443:dbl)
    n298 = local read "stop"() -> (w446:bool)
    n299 = local read "Disp Data"() -> (w449:cluster{"queue out":refnum<queue>, dbl, dbl}[])
    n300 = Wait (ms)(milliseconds to wait=w443) -> ()  [unwired: 1 out]
    n301 = Index Array(array=w449, index="Display Channel") -> (element=w447:cluster{"queue out":refnum<queue>, dbl, dbl})
    n302 = Unbundle(w447) -> (w444:dbl)  [unwired: 2 out]
    "DisplayBarActivation" <- w444
    "DisplayActivation" <- w444
    n303 = call "BarDisplay2Var.vi"("Activation Percentage"=w444, "Target Percentage"="Target Percentage") -> ()  [unwired: 10 in]
    n304 = local read "State"() -> (w445:T1)
    n305 = case shown="\"Trial In Progress\"" w445 {
      tunnel: w444 -> [_ w453 _]
      frame "No Save", Default {
      }
      frame "Trial In Progress" {
        n306 = Format Into String(w453) -> (resulting string=w456:string)  [unwired: 3 in, 1 out]
        n307 = Get Date/Time In Seconds() -> (seconds since 1Jan1904=w454:timestamp)
        n308 = Format Date/Time String(time format string (%c)="%m/%d/%Y, %H:%M:%S%3u", seconds (now)=w454) -> (date/time string=w455:string)  [unwired: 1 in]
        n309 = Build Array(w456, w455) -> (w457:string[])
        n310 = Build Array(w457) -> (w458:string[][])
        n311 = call-poly <vilib>:"Write Delimited Spreadsheet.vi"("file path (dialog if empty)"="trial display data", "2D data"=w458, "append to file? (new file:F)"=TRUE, "delimiter (\\t)"=", " ("delimiter (\\t)")) -> ()  [unwired: 10 in, 2 out]
      }
      frame "Acquiring Max" {
      }
    }
  }
